vi " oef14.3.vi"() -> ()   [LabVIEW 2021]
uses:
  <vilib>/express/express arith-compare/Formula/XNode/ExpressFormulaBlockNode.xnode
panel:
  out "Waveform Graph":dbl[][](graph)
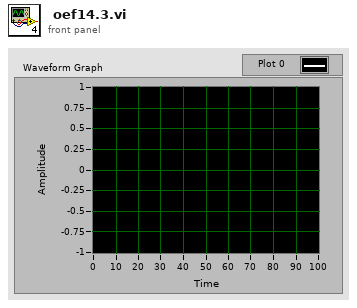
[diagram p1: front panel]
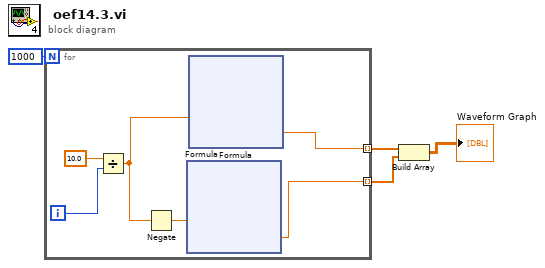
[diagram p0: block diagram]
diagram:
  n1 = for {
    N: 1000 -> [_]
    tunnel: [w10] -> w2 mode=indexing
    tunnel: [w5] -> w3 mode=indexing
    i -> [w8]
    n2 = Divide(x=10.0, y=w8) -> (x/y=w6:dbl)
    n3 = Negate(x=w6) -> (-x=w7:dbl)
    n4 = xnode "Formula"("X1"=w7) -> ("Result"=w5:dbl)  [unwired: 1 in, 1 out]
    n5 = xnode "Formula"("X1"=w6) -> ("Result"=w10:dbl)  [unwired: 1 in, 1 out]
  }
  n6 = Build Array(w2, w3) -> (→"Waveform Graph":dbl[][])
